vi "changing file names.vi"() -> ()   [LabVIEW 2013]
panel:
  out "stripped path":path
  out "name":string
  in  "Auto Folder Path":path=path "E:/Scrubbing/Auto"
  out "size(s)":i32
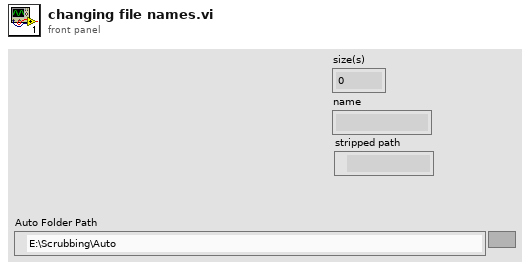
[diagram p1: front panel]
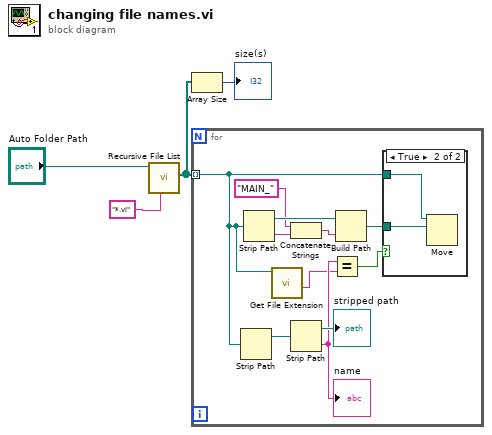
[diagram p0: block diagram]
diagram:
  n1 = call <vilib>:"Recursive File List.vi"("pattern"="*.vi", "Folder Path"="Auto Folder Path") -> ("All Files in Dir"=w1:path[])  [unwired: 5 in, 4 out]
  n2 = Array Size(array=w1) -> (size(s)=→"size(s)":i32)
  n3 = for {
    tunnel: w1 -> [w6] mode=indexing
    n4 = Strip Path(path=w6) -> (stripped path=w11:path)  [unwired: 1 out]
    n5 = Strip Path(path=w6) -> (stripped path=w14:path, name=w8:string)
    n6 = call <vilib>:"Get File Extension.vi"("file"=w6) -> ("filename without extension"=w5:string)  [unwired: 7 in, 3 out]
    n7 = Concatenate Strings("MAIN_" ("string"), w8) -> (w15:string)
    n8 = Strip Path(path=w11) -> (stripped path=→"stripped path":path, name=w9:string)
    "name" <- w9
    n9 = Equal?(x=w9, y=w5) -> (x = y?=w7:bool)
    n10 = Build Path(base path=w14, name or relative path=w15) -> (appended path=w12:path)
    n11 = case shown="True" w7 {
      tunnel: w6 -> [_ w17]
      tunnel: w12 -> [_ w16]
      frame False {
      }
      frame True {
        n12 = Move(source path=w17, 10:w16) -> ()  [unwired: 3 in, 3 out]
      }
    }
  }
